vi "KeyValue Pairs to Query.vi"(11 "Query":cluster{"argument":string, "value":string}[](array[cluster])) -> (3 "query":string)   [LabVIEW 2013, in "openURI.lvlib"]
uses:
  openURI.lvlib
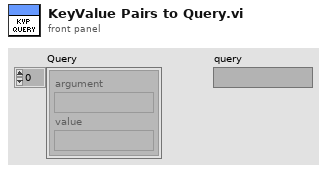
[diagram p1: front panel]
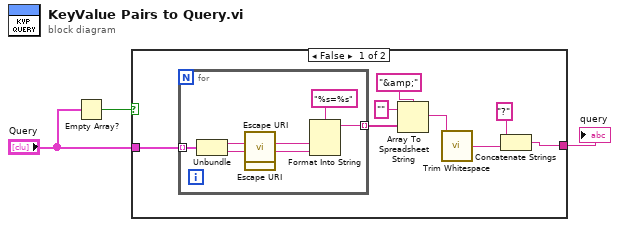
[diagram p0: block diagram]
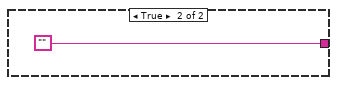
[diagram p2: hidden frame]
diagram:
  n1 = Empty Array?(array="Query") -> (empty?=w3:bool)
  n2 = case shown="False" w3 {
    tunnel: "Query" -> [w11 _]
    tunnel: [w4 ""] -> w1
    frame False {
      n3 = for {
        tunnel: w11 -> [w18] mode=indexing
        tunnel: [w16] -> w10 mode=indexing
        n4 = Unbundle(w18) -> ("argument"=w15:string, "value"=w13:string)
        n5 = call "Escape URI.vi"("URI"=w15) -> ("Escaped URI"=w14:string)  [unwired: 10 in]
        n6 = call "Escape URI.vi"("URI"=w13) -> ("Escaped URI"=w12:string)  [unwired: 10 in]
        n7 = Format Into String(format string="%s=%s", w14, w12) -> (resulting string=w16:string)  [unwired: 2 in, 1 out]
      }
      n8 = Array To Spreadsheet String(delimiter (Tab)="&amp;", array=w10, 3:"" ("format string")) -> (spreadsheet string=w7:string)
      n9 = call <vilib>:"Trim Whitespace.vi"("string"=w7) -> ("trimmed string"=w5:string)  [unwired: 1 in]
      n10 = Concatenate Strings("?" ("t"), w5) -> (w4:string)
    }
    frame True {
    }
  }
  "query" <- w1
